vi "WLM Start and wait.vi"(8 "error in (no error)":errorcluster, 10 "command (show)":enum16{"show", "hide", "exit"}(ring)) -> (0 "error out":errorcluster)   [LabVIEW 2009]
doc: "Starts the wavelength meter server and waits until it is done initializing."
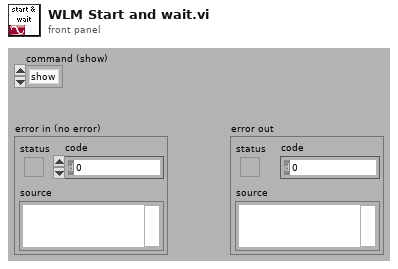
[diagram p1: front panel]
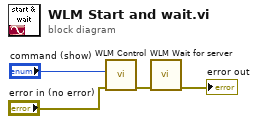
[diagram p0: block diagram]
diagram:
  n1 = call "WLM Control.vi"("error in (no error)"="error in (no error)", "command"="command (show)") -> ("error out"=w4:errorcluster)  [unwired: 9 out]
  n2 = call "WLM Wait for server.vi"("error in (no error)"=w4) -> ("error out"=→"error out":errorcluster)  [unwired: 1 in, 9 out]
